vi "Read Param.vi"(8 "error in (no error)":errorcluster, 11 "MB_TCP in":refnum<class "Modbus Master CR.lvclass">) -> (0 "error out":errorcluster, 2 "Param":refnum<class "MB Param.lvclass">, 3 "MB_TCP out":refnum<class "Modbus Master CR.lvclass">)   [LabVIEW 2021, in "Modbus Master CR.lvclass"]
uses:
  Modbus Master CR.lvclass
  MB Param/MB Param/MB Param.lvclass
  Modbus Master CR.lvclass/Modbus Master CR.ctl
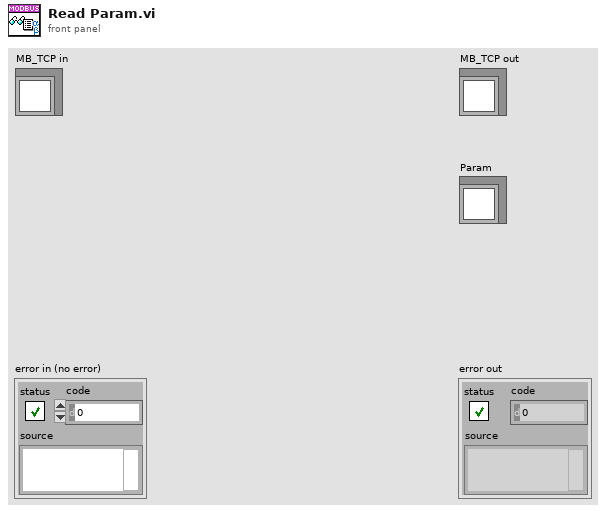
[diagram p1: front panel]
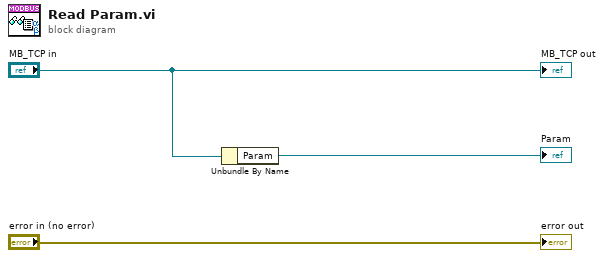
[diagram p0: block diagram]
diagram:
  n1 = Unbundle By Name("MB_TCP in") -> ("Param"=→"Param":refnum<class "MB Param.lvclass">)
  "error out" <- "error in (no error)"
  "MB_TCP out" <- "MB_TCP in"
